vi "convert pixel values to real world.vi"() -> ()   [LabVIEW 2013]
uses:
  <vilib>/vision/Calibration.llb/Calibration Reference Points.ctl
  <vilib>/vision/NI_Vision_Development_Module.lvlib
panel:
  out "manual bottom FangYang vs Ueda":T1[](array[typedef])=[{"X"=365.0, "Y"=447.0}, {"X"=363.0, "Y"=447.0}, {"X"=365.0, "Y"=440.0}, {"X"=360.0, "Y"=440.0}, {"X"=351.0, "Y"=442.0}, {"X"=350.0, "Y"=445.0}, {"X"=347.0, "Y"=443.0}, {"X"=352.0, "Y"=437.0}, {"X"=364.0, "Y"=426.0}, {"X"=392.0, "Y"=419.0}, {"X"=422.0, "Y"=411.0}, {"X"=431.0, "Y"=406.0}, {"X"=441.0, "Y"=402.0}, {"X"=445.0, "Y"=405.0}, {"X"=447.0, "Y"=409.0}, {"X"=452.0, "Y"=407.0}, {"X"=444.0, "Y"=409.0}, {"X"=425.0, "Y"=408.0}, {"X"=410.0, "Y"=416.0}, {"X"=405.0, "Y"=422.0}, {"X"=400.0, "Y"=430.0}, {"X"=400.0, "Y"=423.0}, {"X"=421.0, "Y"=411.0}, {"X"=444.0, "Y"=405.0}, {"X"=451.0, "Y"=407.0}, {"X"=457.0, "Y"=407.0}, {"X"=462.0, "Y"=407.0}, {"X"=463.0, "Y"=406.0}, {"X"=454.0, "Y"=405.0}, {"X"=446.0, "Y"=408.0}, {"X"=435.0, "Y"=414.0}, {"X"=416.0, "Y"=423.0}, {"X"=406.0, "Y"=428.0}, {"X"=399.0, "Y"=438.0}, {"X"=392.0, "Y"=448.0}, {"X"=391.0, "Y"=450.0}, {"X"=387.0, "Y"=448.0}, {"X"=381.0, "Y"=453.0}, {"X"=376.0, "Y"=467.0}, {"X"=370.0, "Y"=469.0}, {"X"=377.0, "Y"=470.0}, {"X"=391.0, "Y"=467.0}, {"X"=412.0, "Y"=468.0}, {"X"=422.0, "Y"=470.0}, {"X"=425.0, "Y"=469.0}, {"X"=426.0, "Y"=466.0}, {"X"=413.0, "Y"=467.0}, {"X"=402.0, "Y"=456.0}, {"X"=384.0, "Y"=452.0}, {"X"=361.0, "Y"=451.0}, {"X"=363.0, "Y"=451.0}, {"X"=353.0, "Y"=456.0}, {"X"=351.0, "Y"=457.0}, {"X"=337.0, "Y"=463.0}, {"X"=324.0, "Y"=475.0}, {"X"=329.0, "Y"=482.0}, {"X"=330.0, "Y"=498.0}, {"X"=333.0, "Y"=505.0}, {"X"=332.0, "Y"=519.0}, {"X"=331.0, "Y"=530.0}, {"X"=328.0, "Y"=526.0}, {"X"=328.0, "Y"=523.0}, {"X"=322.0, "Y"=528.0}, {"X"=316.0, "Y"=530.0}, {"X"=312.0, "Y"=524.0}, {"X"=300.0, "Y"=512.0}, {"X"=296.0, "Y"=507.0}, {"X"=297.0, "Y"=504.0}, {"X"=300.0, "Y"=489.0}, {"X"=300.0, "Y"=484.0}, {"X"=306.0, "Y"=479.0}, {"X"=306.0, "Y"=475.0}, {"X"=306.0, "Y"=466.0}, {"X"=307.0, "Y"=452.0}, {"X"=294.0, "Y"=442.0}, {"X"=266.0, "Y"=436.0}, {"X"=237.0, "Y"=417.0}, {"X"=215.0, "Y"=412.0}, {"X"=208.0, "Y"=420.0}, {"X"=205.0, "Y"=413.0}, {"X"=205.0, "Y"=410.0}, {"X"=206.0, "Y"=413.0}, {"X"=225.0, "Y"=422.0}, {"X"=246.0, "Y"=432.0}, {"X"=249.0, "Y"=435.0}, {"X"=258.0, "Y"=442.0}, {"X"=274.0, "Y"=448.0}, {"X"=285.0, "Y"=455.0}, {"X"=296.0, "Y"=458.0}, {"X"=297.0, "Y"=457.0}, {"X"=283.0, "Y"=455.0}, {"X"=272.0, "Y"=459.0}, {"X"=257.0, "Y"=462.0}, {"X"=250.0, "Y"=470.0}, {"X"=238.0, "Y"=474.0}, {"X"=232.0, "Y"=487.0}, {"X"=223.0, "Y"=494.0}, {"X"=219.0, "Y"=499.0}, {"X"=221.0, "Y"=512.0}, {"X"=214.0, "Y"=514.0}, {"X"=216.0, "Y"=508.0}, {"X"=230.0, "Y"=496.0}, {"X"=245.0, "Y"=485.0}, {"X"=258.0, "Y"=484.0}, {"X"=287.0, "Y"=471.0}, {"X"=310.0, "Y"=461.0}, {"X"=315.0, "Y"=456.0}, {"X"=324.0, "Y"=449.0}, {"X"=330.0, "Y"=437.0}, {"X"=340.0, "Y"=429.0}, {"X"=347.0, "Y"=438.0}, {"X"=354.0, "Y"=446.0}, {"X"=353.0, "Y"=449.0}, {"X"=359.0, "Y"=451.0}, {"X"=368.0, "Y"=445.0}, {"X"=258.0, "Y"=444.0}, {"X"=262.0, "Y"=440.0}, {"X"=272.0, "Y"=434.0}, {"X"=274.0, "Y"=426.0}, {"X"=277.0, "Y"=423.0}, {"X"=276.0, "Y"=426.0}, {"X"=277.0, "Y"=423.0}, {"X"=282.0, "Y"=423.0}, {"X"=285.0, "Y"=426.0}, {"X"=288.0, "Y"=430.0}, {"X"=292.0, "Y"=438.0}, {"X"=293.0, "Y"=446.0}, {"X"=290.0, "Y"=454.0}, {"X"=293.0, "Y"=456.0}, {"X"=299.0, "Y"=464.0}, {"X"=303.0, "Y"=464.0}, {"X"=300.0, "Y"=464.0}, {"X"=294.0, "Y"=464.0}, {"X"=289.0, "Y"=462.0}, {"X"=273.0, "Y"=460.0}, {"X"=245.0, "Y"=457.0}, {"X"=213.0, "Y"=463.0}, {"X"=205.0, "Y"=465.0}, {"X"=205.0, "Y"=463.0}, {"X"=214.0, "Y"=462.0}, {"X"=245.0, "Y"=460.0}, {"X"=287.0, "Y"=466.0}, {"X"=303.0, "Y"=463.0}, {"X"=315.0, "Y"=457.0}, {"X"=335.0, "Y"=469.0}, {"X"=352.0, "Y"=471.0}, {"X"=361.0, "Y"=465.0}, {"X"=366.0, "Y"=466.0}, {"X"=370.0, "Y"=463.0}, {"X"=376.0, "Y"=467.0}, {"X"=373.0, "Y"=466.0}, {"X"=377.0, "Y"=473.0}, {"X"=376.0, "Y"=471.0}, {"X"=358.0, "Y"=474.0}, {"X"=339.0, "Y"=475.0}, {"X"=420.0, "Y"=441.0}, {"X"=420.0, "Y"=443.0}, {"X"=420.0, "Y"=443.0}, {"X"=424.0, "Y"=435.0}, {"X"=431.0, "Y"=430.0}, {"X"=426.0, "Y"=426.0}, {"X"=427.0, "Y"=427.0}, {"X"=425.0, "Y"=425.0}, {"X"=423.0, "Y"=424.0}, {"X"=415.0, "Y"=430.0}, {"X"=417.0, "Y"=432.0}, {"X"=415.0, "Y"=438.0}, {"X"=410.0, "Y"=441.0}, {"X"=399.0, "Y"=450.0}, {"X"=389.0, "Y"=458.0}, {"X"=388.0, "Y"=459.0}, {"X"=400.0, "Y"=461.0}, {"X"=412.0, "Y"=463.0}, {"X"=413.0, "Y"=458.0}, {"X"=413.0, "Y"=458.0}, {"X"=416.0, "Y"=458.0}, {"X"=420.0, "Y"=460.0}, {"X"=419.0, "Y"=459.0}, {"X"=402.0, "Y"=459.0}, {"X"=395.0, "Y"=460.0}, {"X"=394.0, "Y"=459.0}, {"X"=396.0, "Y"=454.0}, {"X"=397.0, "Y"=452.0}, {"X"=396.0, "Y"=451.0}, {"X"=401.0, "Y"=454.0}, {"X"=408.0, "Y"=442.0}, {"X"=410.0, "Y"=428.0}, {"X"=411.0, "Y"=417.0}, {"X"=404.0, "Y"=402.0}, {"X"=405.0, "Y"=403.0}, {"X"=404.0, "Y"=405.0}, {"X"=396.0, "Y"=402.0}, {"X"=387.0, "Y"=406.0}, {"X"=382.0, "Y"=408.0}, {"X"=378.0, "Y"=413.0}, {"X"=361.0, "Y"=417.0}, {"X"=346.0, "Y"=433.0}, {"X"=335.0, "Y"=443.0}, {"X"=329.0, "Y"=445.0}, {"X"=317.0, "Y"=452.0}, {"X"=313.0, "Y"=457.0}, {"X"=312.0, "Y"=465.0}, {"X"=309.0, "Y"=467.0}, {"X"=305.0, "Y"=469.0}, {"X"=298.0, "Y"=463.0}, {"X"=292.0, "Y"=463.0}, {"X"=267.0, "Y"=466.0}, {"X"=267.0, "Y"=464.0}, {"X"=266.0, "Y"=467.0}, {"X"=268.0, "Y"=465.0}, {"X"=284.0, "Y"=467.0}, {"X"=296.0, "Y"=464.0}, {"X"=303.0, "Y"=466.0}, {"X"=310.0, "Y"=466.0}, {"X"=318.0, "Y"=464.0}, {"X"=327.0, "Y"=467.0}, {"X"=322.0, "Y"=466.0}, {"X"=318.0, "Y"=462.0}, {"X"=297.0, "Y"=465.0}, {"X"=263.0, "Y"=468.0}, {"X"=222.0, "Y"=468.0}, {"X"=174.0, "Y"=472.0}, {"X"=142.0, "Y"=470.0}, {"X"=130.0, "Y"=467.0}, {"X"=131.0, "Y"=467.0}, {"X"=157.0, "Y"=461.0}, {"X"=177.0, "Y"=459.0}, {"X"=207.0, "Y"=458.0}, {"X"=248.0, "Y"=459.0}, {"X"=276.0, "Y"=464.0}, {"X"=300.0, "Y"=463.0}, {"X"=318.0, "Y"=457.0}, {"X"=257.0, "Y"=443.0}, {"X"=260.0, "Y"=444.0}, {"X"=260.0, "Y"=439.0}, {"X"=263.0, "Y"=435.0}, {"X"=268.0, "Y"=424.0}, {"X"=275.0, "Y"=426.0}, {"X"=281.0, "Y"=424.0}, {"X"=278.0, "Y"=415.0}, {"X"=286.0, "Y"=421.0}, {"X"=283.0, "Y"=422.0}, {"X"=289.0, "Y"=416.0}, {"X"=289.0, "Y"=417.0}, {"X"=293.0, "Y"=420.0}, {"X"=290.0, "Y"=423.0}, {"X"=295.0, "Y"=423.0}, {"X"=304.0, "Y"=430.0}, {"X"=304.0, "Y"=441.0}, {"X"=318.0, "Y"=454.0}, {"X"=325.0, "Y"=464.0}, {"X"=334.0, "Y"=469.0}, {"X"=360.0, "Y"=488.0}, {"X"=387.0, "Y"=497.0}, {"X"=409.0, "Y"=511.0}, {"X"=428.0, "Y"=520.0}, {"X"=426.0, "Y"=519.0}, {"X"=422.0, "Y"=514.0}, {"X"=406.0, "Y"=509.0}, {"X"=402.0, "Y"=506.0}, {"X"=402.0, "Y"=502.0}, {"X"=402.0, "Y"=491.0}, {"X"=398.0, "Y"=478.0}, {"X"=394.0, "Y"=471.0}, {"X"=375.0, "Y"=463.0}, {"X"=372.0, "Y"=470.0}, {"X"=375.0, "Y"=473.0}, {"X"=374.0, "Y"=475.0}, {"X"=395.0, "Y"=478.0}, {"X"=425.0, "Y"=485.0}, {"X"=458.0, "Y"=501.0}, {"X"=492.0, "Y"=510.0}, {"X"=503.0, "Y"=518.0}, {"X"=492.0, "Y"=514.0}, {"X"=474.0, "Y"=508.0}, {"X"=459.0, "Y"=499.0}, {"X"=449.0, "Y"=502.0}, {"X"=435.0, "Y"=492.0}, {"X"=414.0, "Y"=490.0}, {"X"=385.0, "Y"=473.0}, {"X"=365.0, "Y"=466.0}, {"X"=338.0, "Y"=464.0}, {"X"=329.0, "Y"=464.0}, {"X"=330.0, "Y"=469.0}, {"X"=334.0, "Y"=476.0}, {"X"=348.0, "Y"=483.0}, {"X"=379.0, "Y"=487.0}, {"X"=405.0, "Y"=495.0}, {"X"=442.0, "Y"=501.0}, {"X"=466.0, "Y"=512.0}, {"X"=476.0, "Y"=515.0}, {"X"=474.0, "Y"=515.0}, {"X"=452.0, "Y"=502.0}, {"X"=435.0, "Y"=497.0}, {"X"=437.0, "Y"=499.0}, {"X"=426.0, "Y"=491.0}, {"X"=415.0, "Y"=481.0}, {"X"=407.0, "Y"=469.0}, {"X"=398.0, "Y"=466.0}, {"X"=384.0, "Y"=465.0}, {"X"=377.0, "Y"=466.0}, {"X"=363.0, "Y"=467.0}, {"X"=329.0, "Y"=475.0}, {"X"=305.0, "Y"=482.0}, {"X"=281.0, "Y"=492.0}, {"X"=252.0, "Y"=507.0}, {"X"=231.0, "Y"=504.0}, {"X"=212.0, "Y"=508.0}, {"X"=203.0, "Y"=516.0}, {"X"=189.0, "Y"=515.0}, {"X"=196.0, "Y"=511.0}, {"X"=221.0, "Y"=496.0}, {"X"=229.0, "Y"=491.0}, {"X"=227.0, "Y"=488.0}, {"X"=223.0, "Y"=483.0}, {"X"=224.0, "Y"=473.0}, {"X"=429.0, "Y"=442.0}, {"X"=430.0, "Y"=440.0}, {"X"=428.0, "Y"=432.0}, {"X"=431.0, "Y"=434.0}, {"X"=425.0, "Y"=430.0}, {"X"=419.0, "Y"=430.0}, {"X"=411.0, "Y"=429.0}, {"X"=411.0, "Y"=430.0}, {"X"=394.0, "Y"=435.0}, {"X"=377.0, "Y"=438.0}, {"X"=357.0, "Y"=447.0}, {"X"=346.0, "Y"=450.0}, {"X"=329.0, "Y"=448.0}, {"X"=319.0, "Y"=458.0}, {"X"=303.0, "Y"=460.0}, {"X"=306.0, "Y"=458.0}, {"X"=285.0, "Y"=459.0}, {"X"=262.0, "Y"=460.0}, {"X"=243.0, "Y"=471.0}, {"X"=222.0, "Y"=481.0}, {"X"=201.0, "Y"=484.0}, {"X"=184.0, "Y"=493.0}, {"X"=170.0, "Y"=504.0}, {"X"=160.0, "Y"=512.0}, {"X"=147.0, "Y"=519.0}, {"X"=155.0, "Y"=519.0}, {"X"=180.0, "Y"=512.0}, {"X"=206.0, "Y"=505.0}, {"X"=213.0, "Y"=501.0}, {"X"=226.0, "Y"=489.0}, {"X"=243.0, "Y"=482.0}, {"X"=255.0, "Y"=475.0}, {"X"=260.0, "Y"=469.0}, {"X"=274.0, "Y"=464.0}, {"X"=285.0, "Y"=466.0}, {"X"=280.0, "Y"=463.0}, {"X"=271.0, "Y"=464.0}, {"X"=247.0, "Y"=464.0}, {"X"=225.0, "Y"=473.0}, {"X"=218.0, "Y"=485.0}, {"X"=197.0, "Y"=496.0}, {"X"=191.0, "Y"=485.0}, {"X"=183.0, "Y"=496.0}, {"X"=188.0, "Y"=500.0}, {"X"=166.0, "Y"=520.0}, {"X"=170.0, "Y"=514.0}, {"X"=172.0, "Y"=512.0}, {"X"=184.0, "Y"=508.0}, {"X"=200.0, "Y"=501.0}, {"X"=241.0, "Y"=486.0}, {"X"=271.0, "Y"=473.0}, {"X"=326.0, "Y"=446.0}, {"X"=335.0, "Y"=448.0}, {"X"=334.0, "Y"=446.0}, {"X"=360.0, "Y"=444.0}, {"X"=375.0, "Y"=447.0}, {"X"=380.0, "Y"=443.0}, {"X"=386.0, "Y"=430.0}, {"X"=386.0, "Y"=424.0}, {"X"=389.0, "Y"=407.0}, {"X"=385.0, "Y"=400.0}, {"X"=387.0, "Y"=396.0}, {"X"=381.0, "Y"=400.0}, {"X"=380.0, "Y"=404.0}, {"X"=379.0, "Y"=407.0}, {"X"=355.0, "Y"=423.0}, {"X"=340.0, "Y"=430.0}, {"X"=331.0, "Y"=437.0}, {"X"=317.0, "Y"=439.0}, {"X"=308.0, "Y"=447.0}, {"X"=284.0, "Y"=454.0}, {"X"=279.0, "Y"=456.0}, {"X"=266.0, "Y"=458.0}, {"X"=262.0, "Y"=459.0}, {"X"=258.0, "Y"=459.0}, {"X"=237.0, "Y"=452.0}, {"X"=231.0, "Y"=449.0}, {"X"=239.0, "Y"=448.0}, {"X"=250.0, "Y"=451.0}, {"X"=264.0, "Y"=450.0}, {"X"=290.0, "Y"=450.0}, {"X"=315.0, "Y"=449.0}, {"X"=329.0, "Y"=453.0}, {"X"=340.0, "Y"=452.0}, {"X"=363.0, "Y"=447.0}, {"X"=382.0, "Y"=432.0}, {"X"=396.0, "Y"=421.0}, {"X"=404.0, "Y"=408.0}, {"X"=408.0, "Y"=407.0}, {"X"=420.0, "Y"=401.0}, {"X"=416.0, "Y"=395.0}, {"X"=418.0, "Y"=400.0}, {"X"=413.0, "Y"=403.0}, {"X"=397.0, "Y"=416.0}, {"X"=393.0, "Y"=418.0}, {"X"=384.0, "Y"=427.0}, {"X"=382.0, "Y"=431.0}, {"X"=380.0, "Y"=435.0}, {"X"=381.0, "Y"=445.0}, {"X"=388.0, "Y"=450.0}, {"X"=382.0, "Y"=460.0}, {"X"=400.0, "Y"=455.0}, {"X"=436.0, "Y"=457.0}, {"X"=456.0, "Y"=449.0}, {"X"=468.0, "Y"=450.0}, {"X"=477.0, "Y"=450.0}, {"X"=474.0, "Y"=448.0}, {"X"=461.0, "Y"=450.0}, {"X"=457.0, "Y"=451.0}, {"X"=451.0, "Y"=445.0}, {"X"=436.0, "Y"=444.0}, {"X"=414.0, "Y"=446.0}, {"X"=391.0, "Y"=445.0}, {"X"=372.0, "Y"=453.0}, {"X"=364.0, "Y"=447.0}, {"X"=363.0, "Y"=454.0}, {"X"=358.0, "Y"=464.0}, {"X"=358.0, "Y"=472.0}, {"X"=373.0, "Y"=484.0}, {"X"=396.0, "Y"=493.0}, {"X"=415.0, "Y"=477.0}, {"X"=439.0, "Y"=502.0}, {"X"=472.0, "Y"=519.0}, {"X"=508.0, "Y"=541.0}, {"X"=497.0, "Y"=529.0}, {"X"=486.0, "Y"=519.0}, {"X"=471.0, "Y"=511.0}, {"X"=452.0, "Y"=501.0}, {"X"=440.0, "Y"=488.0}, {"X"=428.0, "Y"=475.0}, {"X"=404.0, "Y"=462.0}, {"X"=393.0, "Y"=441.0}, {"X"=379.0, "Y"=433.0}, {"X"=381.0, "Y"=437.0}, {"X"=383.0, "Y"=432.0}, {"X"=376.0, "Y"=428.0}, {"X"=370.0, "Y"=429.0}, {"X"=364.0, "Y"=431.0}, {"X"=369.0, "Y"=438.0}, {"X"=364.0, "Y"=442.0}, {"X"=363.0, "Y"=447.0}, {"X"=360.0, "Y"=450.0}, {"X"=360.0, "Y"=457.0}, {"X"=370.0, "Y"=461.0}, {"X"=374.0, "Y"=466.0}, {"X"=371.0, "Y"=466.0}, {"X"=360.0, "Y"=461.0}, {"X"=332.0, "Y"=465.0}, {"X"=299.0, "Y"=453.0}, {"X"=266.0, "Y"=435.0}, {"X"=250.0, "Y"=439.0}, {"X"=236.0, "Y"=435.0}, {"X"=229.0, "Y"=424.0}, {"X"=228.0, "Y"=431.0}, {"X"=232.0, "Y"=440.0}, {"X"=235.0, "Y"=447.0}, {"X"=252.0, "Y"=452.0}, {"X"=265.0, "Y"=462.0}, {"X"=275.0, "Y"=463.0}, {"X"=266.0, "Y"=465.0}, {"X"=269.0, "Y"=466.0}, {"X"=270.0, "Y"=465.0}, {"X"=263.0, "Y"=463.0}, {"X"=266.0, "Y"=467.0}, {"X"=268.0, "Y"=464.0}, {"X"=287.0, "Y"=461.0}, {"X"=312.0, "Y"=460.0}, {"X"=334.0, "Y"=466.0}, {"X"=339.0, "Y"=462.0}, {"X"=342.0, "Y"=463.0}, {"X"=329.0, "Y"=469.0}, {"X"=304.0, "Y"=477.0}, {"X"=290.0, "Y"=489.0}, {"X"=266.0, "Y"=493.0}, {"X"=235.0, "Y"=493.0}, {"X"=215.0, "Y"=498.0}, {"X"=200.0, "Y"=509.0}, {"X"=170.0, "Y"=522.0}, {"X"=166.0, "Y"=526.0}, {"X"=175.0, "Y"=521.0}, {"X"=203.0, "Y"=501.0}, {"X"=232.0, "Y"=491.0}, {"X"=256.0, "Y"=495.0}, {"X"=259.0, "Y"=481.0}, {"X"=254.0, "Y"=469.0}, {"X"=251.0, "Y"=449.0}, {"X"=240.0, "Y"=443.0}, {"X"=228.0, "Y"=434.0}, {"X"=224.0, "Y"=422.0}, {"X"=219.0, "Y"=413.0}, {"X"=207.0, "Y"=413.0}, {"X"=419.0, "Y"=440.0}, {"X"=422.0, "Y"=437.0}, {"X"=416.0, "Y"=436.0}, {"X"=429.0, "Y"=444.0}, {"X"=436.0, "Y"=452.0}, {"X"=437.0, "Y"=457.0}, {"X"=449.0, "Y"=468.0}, {"X"=460.0, "Y"=483.0}, {"X"=468.0, "Y"=496.0}, {"X"=478.0, "Y"=508.0}, {"X"=467.0, "Y"=503.0}, {"X"=438.0, "Y"=493.0}, {"X"=434.0, "Y"=496.0}, {"X"=427.0, "Y"=491.0}, {"X"=416.0, "Y"=481.0}, {"X"=402.0, "Y"=473.0}, {"X"=399.0, "Y"=469.0}, {"X"=405.0, "Y"=458.0}, {"X"=394.0, "Y"=446.0}, {"X"=374.0, "Y"=435.0}, {"X"=359.0, "Y"=429.0}, {"X"=350.0, "Y"=422.0}, {"X"=347.0, "Y"=421.0}, {"X"=338.0, "Y"=426.0}, {"X"=329.0, "Y"=426.0}, {"X"=327.0, "Y"=427.0}, {"X"=326.0, "Y"=426.0}, {"X"=340.0, "Y"=433.0}, {"X"=345.0, "Y"=432.0}, {"X"=379.0, "Y"=421.0}, {"X"=403.0, "Y"=415.0}, {"X"=403.0, "Y"=419.0}, {"X"=411.0, "Y"=413.0}, {"X"=409.0, "Y"=404.0}, {"X"=413.0, "Y"=391.0}, {"X"=403.0, "Y"=377.0}, {"X"=405.0, "Y"=377.0}, {"X"=409.0, "Y"=370.0}, {"X"=412.0, "Y"=366.0}, {"X"=397.0, "Y"=370.0}, {"X"=376.0, "Y"=376.0}, {"X"=366.0, "Y"=377.0}, {"X"=348.0, "Y"=376.0}, {"X"=0.0, "Y"=0.0}] {"Y" format="%.2f"; "X" format="%.2f"}
  in  "auto top FangYang vs Ueda":cluster{"Numeric":dbl, "Numeric":dbl}[](array[cluster])=[{"Numeric"=0.0, "Numeric"=0.0}, {"Numeric"=288.0, "Numeric"=288.0}, {"Numeric"=285.0, "Numeric"=292.0}, {"Numeric"=286.0, "Numeric"=308.0}, {"Numeric"=292.0, "Numeric"=309.0}, {"Numeric"=307.0, "Numeric"=306.0}, {"Numeric"=311.0, "Numeric"=298.0}, {"Numeric"=316.0, "Numeric"=299.0}, {"Numeric"=324.0, "Numeric"=289.0}, {"Numeric"=332.0, "Numeric"=288.0}, {"Numeric"=336.0, "Numeric"=294.0}, {"Numeric"=355.0, "Numeric"=288.0}, {"Numeric"=374.0, "Numeric"=286.0}, {"Numeric"=381.0, "Numeric"=288.0}, {"Numeric"=381.0, "Numeric"=288.0}, {"Numeric"=420.0, "Numeric"=295.0}, {"Numeric"=426.0, "Numeric"=296.0}, {"Numeric"=442.0, "Numeric"=308.0}, {"Numeric"=456.0, "Numeric"=318.0}, {"Numeric"=465.0, "Numeric"=330.0}, {"Numeric"=470.0, "Numeric"=321.0}, {"Numeric"=457.0, "Numeric"=312.0}, {"Numeric"=457.0, "Numeric"=312.0}, {"Numeric"=448.0, "Numeric"=310.0}, {"Numeric"=443.0, "Numeric"=295.0}, {"Numeric"=437.0, "Numeric"=291.0}, {"Numeric"=421.0, "Numeric"=295.0}, {"Numeric"=408.0, "Numeric"=298.0}, {"Numeric"=402.0, "Numeric"=298.0}, {"Numeric"=380.0, "Numeric"=298.0}, {"Numeric"=380.0, "Numeric"=277.0}, {"Numeric"=407.0, "Numeric"=299.0}, {"Numeric"=410.0, "Numeric"=299.0}, {"Numeric"=418.0, "Numeric"=257.0}, {"Numeric"=430.0, "Numeric"=252.0}, {"Numeric"=436.0, "Numeric"=252.0}, {"Numeric"=446.0, "Numeric"=242.0}, {"Numeric"=444.0, "Numeric"=236.0}, {"Numeric"=448.0, "Numeric"=230.0}, {"Numeric"=448.0, "Numeric"=234.0}, {"Numeric"=451.0, "Numeric"=236.0}, {"Numeric"=452.0, "Numeric"=243.0}, {"Numeric"=450.0, "Numeric"=254.0}, {"Numeric"=446.0, "Numeric"=263.0}, {"Numeric"=440.0, "Numeric"=272.0}, {"Numeric"=435.0, "Numeric"=273.0}, {"Numeric"=426.0, "Numeric"=281.0}, {"Numeric"=426.0, "Numeric"=290.0}, {"Numeric"=418.0, "Numeric"=292.0}, {"Numeric"=410.0, "Numeric"=318.0}, {"Numeric"=400.0, "Numeric"=331.0}, {"Numeric"=392.0, "Numeric"=336.0}, {"Numeric"=373.0, "Numeric"=309.0}, {"Numeric"=370.0, "Numeric"=312.0}, {"Numeric"=371.0, "Numeric"=313.0}, {"Numeric"=371.0, "Numeric"=299.0}, {"Numeric"=368.0, "Numeric"=298.0}, {"Numeric"=369.0, "Numeric"=297.0}, {"Numeric"=364.0, "Numeric"=292.0}, {"Numeric"=358.0, "Numeric"=283.0}, {"Numeric"=352.0, "Numeric"=278.0}, {"Numeric"=350.0, "Numeric"=278.0}, {"Numeric"=349.0, "Numeric"=276.0}, {"Numeric"=342.0, "Numeric"=273.0}, {"Numeric"=329.0, "Numeric"=270.0}, {"Numeric"=328.0, "Numeric"=270.0}, {"Numeric"=330.0, "Numeric"=269.0}, {"Numeric"=316.0, "Numeric"=271.0}, {"Numeric"=289.0, "Numeric"=268.0}, {"Numeric"=270.0, "Numeric"=282.0}, {"Numeric"=265.0, "Numeric"=286.0}, {"Numeric"=262.0, "Numeric"=263.0}, {"Numeric"=256.0, "Numeric"=281.0}, {"Numeric"=258.0, "Numeric"=282.0}, {"Numeric"=262.0, "Numeric"=278.0}, {"Numeric"=269.0, "Numeric"=289.0}, {"Numeric"=277.0, "Numeric"=289.0}, {"Numeric"=271.0, "Numeric"=288.0}, {"Numeric"=278.0, "Numeric"=287.0}, {"Numeric"=286.0, "Numeric"=284.0}, {"Numeric"=290.0, "Numeric"=284.0}, {"Numeric"=277.0, "Numeric"=283.0}, {"Numeric"=277.0, "Numeric"=272.0}, {"Numeric"=282.0, "Numeric"=268.0}, {"Numeric"=274.0, "Numeric"=265.0}, {"Numeric"=265.0, "Numeric"=255.0}, {"Numeric"=269.0, "Numeric"=253.0}, {"Numeric"=253.0, "Numeric"=235.0}, {"Numeric"=248.0, "Numeric"=231.0}, {"Numeric"=249.0, "Numeric"=235.0}, {"Numeric"=257.0, "Numeric"=238.0}, {"Numeric"=260.0, "Numeric"=240.0}, {"Numeric"=268.0, "Numeric"=249.0}, {"Numeric"=275.0, "Numeric"=253.0}, {"Numeric"=283.0, "Numeric"=257.0}, {"Numeric"=287.0, "Numeric"=263.0}, {"Numeric"=293.0, "Numeric"=263.0}, {"Numeric"=302.0, "Numeric"=266.0}, {"Numeric"=303.0, "Numeric"=271.0}, {"Numeric"=301.0, "Numeric"=271.0}, {"Numeric"=290.0, "Numeric"=272.0}, {"Numeric"=296.0, "Numeric"=249.0}, {"Numeric"=299.0, "Numeric"=269.0}, {"Numeric"=304.0, "Numeric"=267.0}, {"Numeric"=312.0, "Numeric"=271.0}, {"Numeric"=316.0, "Numeric"=271.0}, {"Numeric"=319.0, "Numeric"=271.0}, {"Numeric"=322.0, "Numeric"=271.0}, {"Numeric"=312.0, "Numeric"=270.0}, {"Numeric"=337.0, "Numeric"=269.0}, {"Numeric"=335.0, "Numeric"=275.0}, {"Numeric"=367.0, "Numeric"=270.0}, {"Numeric"=328.0, "Numeric"=273.0}, {"Numeric"=380.0, "Numeric"=274.0}, {"Numeric"=374.0, "Numeric"=274.0}, {"Numeric"=374.0, "Numeric"=274.0}, {"Numeric"=340.0, "Numeric"=286.0}, {"Numeric"=336.0, "Numeric"=287.0}, {"Numeric"=336.0, "Numeric"=281.0}, {"Numeric"=336.0, "Numeric"=285.0}, {"Numeric"=333.0, "Numeric"=285.0}, {"Numeric"=335.0, "Numeric"=284.0}, {"Numeric"=334.0, "Numeric"=285.0}, {"Numeric"=328.0, "Numeric"=295.0}, {"Numeric"=307.0, "Numeric"=284.0}, {"Numeric"=280.0, "Numeric"=283.0}, {"Numeric"=276.0, "Numeric"=283.0}, {"Numeric"=274.0, "Numeric"=267.0}, {"Numeric"=264.0, "Numeric"=250.0}, {"Numeric"=259.0, "Numeric"=249.0}, {"Numeric"=244.0, "Numeric"=243.0}, {"Numeric"=234.0, "Numeric"=232.0}, {"Numeric"=247.0, "Numeric"=241.0}, {"Numeric"=251.0, "Numeric"=241.0}, {"Numeric"=267.0, "Numeric"=251.0}, {"Numeric"=280.0, "Numeric"=262.0}, {"Numeric"=289.0, "Numeric"=272.0}, {"Numeric"=307.0, "Numeric"=258.0}, {"Numeric"=319.0, "Numeric"=283.0}, {"Numeric"=340.0, "Numeric"=283.0}, {"Numeric"=374.0, "Numeric"=299.0}, {"Numeric"=387.0, "Numeric"=307.0}, {"Numeric"=375.0, "Numeric"=301.0}, {"Numeric"=403.0, "Numeric"=313.0}, {"Numeric"=415.0, "Numeric"=312.0}, {"Numeric"=409.0, "Numeric"=307.0}, {"Numeric"=361.0, "Numeric"=311.0}, {"Numeric"=411.0, "Numeric"=313.0}, {"Numeric"=419.0, "Numeric"=312.0}, {"Numeric"=444.0, "Numeric"=310.0}, {"Numeric"=436.0, "Numeric"=325.0}, {"Numeric"=442.0, "Numeric"=328.0}, {"Numeric"=446.0, "Numeric"=325.0}, {"Numeric"=447.0, "Numeric"=332.0}, {"Numeric"=449.0, "Numeric"=340.0}, {"Numeric"=449.0, "Numeric"=340.0}, {"Numeric"=333.0, "Numeric"=275.0}, {"Numeric"=335.0, "Numeric"=281.0}, {"Numeric"=336.0, "Numeric"=276.0}, {"Numeric"=334.0, "Numeric"=277.0}, {"Numeric"=341.0, "Numeric"=283.0}, {"Numeric"=352.0, "Numeric"=288.0}, {"Numeric"=360.0, "Numeric"=285.0}, {"Numeric"=367.0, "Numeric"=282.0}, {"Numeric"=378.0, "Numeric"=288.0}, {"Numeric"=386.0, "Numeric"=270.0}, {"Numeric"=388.0, "Numeric"=266.0}, {"Numeric"=403.0, "Numeric"=261.0}, {"Numeric"=407.0, "Numeric"=257.0}, {"Numeric"=419.0, "Numeric"=255.0}, {"Numeric"=429.0, "Numeric"=253.0}, {"Numeric"=436.0, "Numeric"=258.0}, {"Numeric"=409.0, "Numeric"=261.0}, {"Numeric"=401.0, "Numeric"=258.0}, {"Numeric"=392.0, "Numeric"=263.0}, {"Numeric"=381.0, "Numeric"=273.0}, {"Numeric"=377.0, "Numeric"=277.0}, {"Numeric"=371.0, "Numeric"=276.0}, {"Numeric"=377.0, "Numeric"=281.0}, {"Numeric"=388.0, "Numeric"=281.0}, {"Numeric"=413.0, "Numeric"=288.0}, {"Numeric"=432.0, "Numeric"=288.0}, {"Numeric"=435.0, "Numeric"=296.0}, {"Numeric"=456.0, "Numeric"=310.0}, {"Numeric"=453.0, "Numeric"=320.0}, {"Numeric"=450.0, "Numeric"=316.0}, {"Numeric"=450.0, "Numeric"=316.0}, {"Numeric"=433.0, "Numeric"=320.0}, {"Numeric"=426.0, "Numeric"=314.0}, {"Numeric"=405.0, "Numeric"=312.0}, {"Numeric"=406.0, "Numeric"=312.0}, {"Numeric"=392.0, "Numeric"=314.0}, {"Numeric"=379.0, "Numeric"=311.0}, {"Numeric"=359.0, "Numeric"=310.0}, {"Numeric"=342.0, "Numeric"=310.0}, {"Numeric"=334.0, "Numeric"=309.0}, {"Numeric"=309.0, "Numeric"=251.0}, {"Numeric"=333.0, "Numeric"=258.0}, {"Numeric"=313.0, "Numeric"=248.0}, {"Numeric"=291.0, "Numeric"=246.0}, {"Numeric"=277.0, "Numeric"=244.0}, {"Numeric"=265.0, "Numeric"=238.0}, {"Numeric"=267.0, "Numeric"=241.0}, {"Numeric"=270.0, "Numeric"=240.0}, {"Numeric"=277.0, "Numeric"=251.0}, {"Numeric"=291.0, "Numeric"=262.0}, {"Numeric"=293.0, "Numeric"=267.0}, {"Numeric"=294.0, "Numeric"=270.0}, {"Numeric"=288.0, "Numeric"=270.0}, {"Numeric"=275.0, "Numeric"=266.0}, {"Numeric"=272.0, "Numeric"=260.0}, {"Numeric"=271.0, "Numeric"=262.0}, {"Numeric"=274.0, "Numeric"=253.0}, {"Numeric"=266.0, "Numeric"=246.0}, {"Numeric"=265.0, "Numeric"=242.0}, {"Numeric"=260.0, "Numeric"=238.0}, {"Numeric"=260.0, "Numeric"=235.0}, {"Numeric"=261.0, "Numeric"=235.0}, {"Numeric"=260.0, "Numeric"=237.0}, {"Numeric"=258.0, "Numeric"=246.0}, {"Numeric"=264.0, "Numeric"=252.0}, {"Numeric"=263.0, "Numeric"=260.0}, {"Numeric"=259.0, "Numeric"=259.0}, {"Numeric"=252.0, "Numeric"=279.0}, {"Numeric"=247.0, "Numeric"=295.0}, {"Numeric"=238.0, "Numeric"=298.0}, {"Numeric"=233.0, "Numeric"=310.0}, {"Numeric"=225.0, "Numeric"=313.0}, {"Numeric"=228.0, "Numeric"=314.0}, {"Numeric"=196.0, "Numeric"=327.0}, {"Numeric"=192.0, "Numeric"=334.0}, {"Numeric"=184.0, "Numeric"=342.0}, {"Numeric"=182.0, "Numeric"=341.0}, {"Numeric"=339.0, "Numeric"=272.0}, {"Numeric"=340.0, "Numeric"=288.0}, {"Numeric"=346.0, "Numeric"=288.0}, {"Numeric"=344.0, "Numeric"=288.0}, {"Numeric"=335.0, "Numeric"=287.0}, {"Numeric"=335.0, "Numeric"=287.0}, {"Numeric"=330.0, "Numeric"=287.0}, {"Numeric"=305.0, "Numeric"=295.0}, {"Numeric"=289.0, "Numeric"=292.0}, {"Numeric"=292.0, "Numeric"=296.0}, {"Numeric"=278.0, "Numeric"=301.0}, {"Numeric"=257.0, "Numeric"=315.0}, {"Numeric"=328.0, "Numeric"=282.0}, {"Numeric"=255.0, "Numeric"=329.0}, {"Numeric"=273.0, "Numeric"=314.0}, {"Numeric"=282.0, "Numeric"=300.0}, {"Numeric"=295.0, "Numeric"=289.0}, {"Numeric"=306.0, "Numeric"=286.0}, {"Numeric"=308.0, "Numeric"=286.0}, {"Numeric"=325.0, "Numeric"=296.0}, {"Numeric"=331.0, "Numeric"=292.0}, {"Numeric"=342.0, "Numeric"=289.0}, {"Numeric"=357.0, "Numeric"=283.0}, {"Numeric"=367.0, "Numeric"=281.0}, {"Numeric"=367.0, "Numeric"=276.0}, {"Numeric"=385.0, "Numeric"=268.0}, {"Numeric"=392.0, "Numeric"=279.0}, {"Numeric"=410.0, "Numeric"=287.0}, {"Numeric"=418.0, "Numeric"=294.0}, {"Numeric"=425.0, "Numeric"=299.0}, {"Numeric"=427.0, "Numeric"=266.0}, {"Numeric"=425.0, "Numeric"=266.0}, {"Numeric"=420.0, "Numeric"=294.0}, {"Numeric"=415.0, "Numeric"=293.0}, {"Numeric"=408.0, "Numeric"=290.0}, {"Numeric"=403.0, "Numeric"=288.0}, {"Numeric"=397.0, "Numeric"=286.0}, {"Numeric"=389.0, "Numeric"=275.0}, {"Numeric"=388.0, "Numeric"=275.0}, {"Numeric"=382.0, "Numeric"=272.0}, {"Numeric"=381.0, "Numeric"=271.0}, {"Numeric"=365.0, "Numeric"=267.0}, {"Numeric"=353.0, "Numeric"=269.0}, {"Numeric"=333.0, "Numeric"=281.0}, {"Numeric"=313.0, "Numeric"=277.0}, {"Numeric"=304.0, "Numeric"=286.0}, {"Numeric"=279.0, "Numeric"=296.0}, {"Numeric"=274.0, "Numeric"=289.0}, {"Numeric"=274.0, "Numeric"=283.0}, {"Numeric"=270.0, "Numeric"=292.0}, {"Numeric"=276.0, "Numeric"=290.0}, {"Numeric"=285.0, "Numeric"=289.0}, {"Numeric"=301.0, "Numeric"=286.0}, {"Numeric"=319.0, "Numeric"=279.0}, {"Numeric"=329.0, "Numeric"=278.0}, {"Numeric"=336.0, "Numeric"=275.0}, {"Numeric"=337.0, "Numeric"=274.0}, {"Numeric"=362.0, "Numeric"=271.0}, {"Numeric"=367.0, "Numeric"=269.0}, {"Numeric"=374.0, "Numeric"=265.0}, {"Numeric"=377.0, "Numeric"=273.0}, {"Numeric"=383.0, "Numeric"=268.0}, {"Numeric"=397.0, "Numeric"=284.0}, {"Numeric"=421.0, "Numeric"=285.0}, {"Numeric"=418.0, "Numeric"=285.0}, {"Numeric"=428.0, "Numeric"=276.0}, {"Numeric"=415.0, "Numeric"=285.0}, {"Numeric"=404.0, "Numeric"=289.0}, {"Numeric"=398.0, "Numeric"=288.0}, {"Numeric"=390.0, "Numeric"=284.0}, {"Numeric"=377.0, "Numeric"=283.0}, {"Numeric"=362.0, "Numeric"=280.0}, {"Numeric"=350.0, "Numeric"=276.0}, {"Numeric"=340.0, "Numeric"=274.0}, {"Numeric"=333.0, "Numeric"=275.0}, {"Numeric"=323.0, "Numeric"=270.0}, {"Numeric"=323.0, "Numeric"=269.0}, {"Numeric"=306.0, "Numeric"=269.0}, {"Numeric"=297.0, "Numeric"=265.0}, {"Numeric"=284.0, "Numeric"=267.0}, {"Numeric"=272.0, "Numeric"=271.0}, {"Numeric"=241.0, "Numeric"=271.0}, {"Numeric"=236.0, "Numeric"=270.0}, {"Numeric"=230.0, "Numeric"=271.0}, {"Numeric"=336.0, "Numeric"=273.0}, {"Numeric"=335.0, "Numeric"=276.0}, {"Numeric"=342.0, "Numeric"=272.0}, {"Numeric"=348.0, "Numeric"=288.0}, {"Numeric"=361.0, "Numeric"=289.0}, {"Numeric"=377.0, "Numeric"=291.0}, {"Numeric"=371.0, "Numeric"=295.0}, {"Numeric"=353.0, "Numeric"=289.0}, {"Numeric"=328.0, "Numeric"=288.0}, {"Numeric"=335.0, "Numeric"=268.0}, {"Numeric"=311.0, "Numeric"=260.0}, {"Numeric"=301.0, "Numeric"=251.0}, {"Numeric"=280.0, "Numeric"=247.0}, {"Numeric"=265.0, "Numeric"=238.0}, {"Numeric"=261.0, "Numeric"=237.0}, {"Numeric"=271.0, "Numeric"=248.0}, {"Numeric"=264.0, "Numeric"=246.0}, {"Numeric"=272.0, "Numeric"=253.0}, {"Numeric"=276.0, "Numeric"=252.0}, {"Numeric"=277.0, "Numeric"=255.0}, {"Numeric"=285.0, "Numeric"=262.0}, {"Numeric"=289.0, "Numeric"=268.0}, {"Numeric"=294.0, "Numeric"=279.0}, {"Numeric"=291.0, "Numeric"=279.0}, {"Numeric"=288.0, "Numeric"=276.0}, {"Numeric"=288.0, "Numeric"=273.0}, {"Numeric"=284.0, "Numeric"=276.0}, {"Numeric"=260.0, "Numeric"=273.0}, {"Numeric"=242.0, "Numeric"=260.0}, {"Numeric"=250.0, "Numeric"=268.0}, {"Numeric"=245.0, "Numeric"=255.0}, {"Numeric"=246.0, "Numeric"=248.0}, {"Numeric"=244.0, "Numeric"=244.0}, {"Numeric"=236.0, "Numeric"=232.0}, {"Numeric"=233.0, "Numeric"=228.0}, {"Numeric"=239.0, "Numeric"=235.0}, {"Numeric"=245.0, "Numeric"=238.0}, {"Numeric"=256.0, "Numeric"=247.0}, {"Numeric"=266.0, "Numeric"=251.0}, {"Numeric"=273.0, "Numeric"=252.0}, {"Numeric"=280.0, "Numeric"=258.0}, {"Numeric"=288.0, "Numeric"=263.0}, {"Numeric"=299.0, "Numeric"=265.0}, {"Numeric"=304.0, "Numeric"=271.0}, {"Numeric"=303.0, "Numeric"=268.0}, {"Numeric"=310.0, "Numeric"=266.0}, {"Numeric"=320.0, "Numeric"=266.0}, {"Numeric"=329.0, "Numeric"=267.0}, {"Numeric"=336.0, "Numeric"=264.0}, {"Numeric"=340.0, "Numeric"=270.0}, {"Numeric"=387.0, "Numeric"=285.0}, {"Numeric"=416.0, "Numeric"=288.0}, {"Numeric"=414.0, "Numeric"=309.0}, {"Numeric"=418.0, "Numeric"=319.0}, {"Numeric"=419.0, "Numeric"=313.0}, {"Numeric"=418.0, "Numeric"=320.0}, {"Numeric"=418.0, "Numeric"=326.0}, {"Numeric"=417.0, "Numeric"=326.0}, {"Numeric"=412.0, "Numeric"=325.0}, {"Numeric"=412.0, "Numeric"=324.0}, {"Numeric"=410.0, "Numeric"=326.0}, {"Numeric"=399.0, "Numeric"=331.0}, {"Numeric"=372.0, "Numeric"=325.0}, {"Numeric"=352.0, "Numeric"=317.0}, {"Numeric"=329.0, "Numeric"=316.0}, {"Numeric"=307.0, "Numeric"=315.0}, {"Numeric"=295.0, "Numeric"=315.0}, {"Numeric"=292.0, "Numeric"=258.0}, {"Numeric"=208.0, "Numeric"=198.0}, {"Numeric"=251.0, "Numeric"=248.0}, {"Numeric"=241.0, "Numeric"=244.0}, {"Numeric"=260.0, "Numeric"=252.0}, {"Numeric"=252.0, "Numeric"=251.0}, {"Numeric"=259.0, "Numeric"=258.0}, {"Numeric"=264.0, "Numeric"=262.0}, {"Numeric"=271.0, "Numeric"=262.0}, {"Numeric"=296.0, "Numeric"=269.0}, {"Numeric"=311.0, "Numeric"=288.0}, {"Numeric"=323.0, "Numeric"=293.0}, {"Numeric"=326.0, "Numeric"=307.0}, {"Numeric"=322.0, "Numeric"=300.0}, {"Numeric"=334.0, "Numeric"=325.0}, {"Numeric"=336.0, "Numeric"=311.0}, {"Numeric"=337.0, "Numeric"=305.0}, {"Numeric"=346.0, "Numeric"=307.0}, {"Numeric"=350.0, "Numeric"=300.0}, {"Numeric"=334.0, "Numeric"=308.0}, {"Numeric"=339.0, "Numeric"=303.0}, {"Numeric"=341.0, "Numeric"=299.0}, {"Numeric"=349.0, "Numeric"=296.0}, {"Numeric"=357.0, "Numeric"=286.0}, {"Numeric"=357.0, "Numeric"=301.0}, {"Numeric"=370.0, "Numeric"=302.0}, {"Numeric"=363.0, "Numeric"=269.0}, {"Numeric"=367.0, "Numeric"=258.0}, {"Numeric"=380.0, "Numeric"=252.0}, {"Numeric"=398.0, "Numeric"=248.0}, {"Numeric"=403.0, "Numeric"=249.0}, {"Numeric"=425.0, "Numeric"=242.0}, {"Numeric"=429.0, "Numeric"=241.0}, {"Numeric"=418.0, "Numeric"=242.0}, {"Numeric"=403.0, "Numeric"=249.0}, {"Numeric"=391.0, "Numeric"=251.0}, {"Numeric"=385.0, "Numeric"=253.0}, {"Numeric"=379.0, "Numeric"=260.0}, {"Numeric"=373.0, "Numeric"=265.0}, {"Numeric"=374.0, "Numeric"=267.0}, {"Numeric"=378.0, "Numeric"=270.0}, {"Numeric"=389.0, "Numeric"=275.0}, {"Numeric"=409.0, "Numeric"=275.0}, {"Numeric"=410.0, "Numeric"=275.0}, {"Numeric"=416.0, "Numeric"=277.0}, {"Numeric"=421.0, "Numeric"=289.0}, {"Numeric"=412.0, "Numeric"=290.0}, {"Numeric"=408.0, "Numeric"=304.0}, {"Numeric"=403.0, "Numeric"=301.0}, {"Numeric"=400.0, "Numeric"=294.0}, {"Numeric"=395.0, "Numeric"=290.0}, {"Numeric"=384.0, "Numeric"=282.0}, {"Numeric"=378.0, "Numeric"=280.0}, {"Numeric"=376.0, "Numeric"=277.0}, {"Numeric"=368.0, "Numeric"=272.0}, {"Numeric"=365.0, "Numeric"=268.0}, {"Numeric"=376.0, "Numeric"=266.0}, {"Numeric"=388.0, "Numeric"=264.0}, {"Numeric"=386.0, "Numeric"=266.0}, {"Numeric"=372.0, "Numeric"=244.0}, {"Numeric"=378.0, "Numeric"=268.0}, {"Numeric"=377.0, "Numeric"=270.0}, {"Numeric"=372.0, "Numeric"=270.0}, {"Numeric"=364.0, "Numeric"=286.0}, {"Numeric"=357.0, "Numeric"=288.0}, {"Numeric"=356.0, "Numeric"=274.0}, {"Numeric"=349.0, "Numeric"=276.0}, {"Numeric"=350.0, "Numeric"=274.0}, {"Numeric"=354.0, "Numeric"=280.0}, {"Numeric"=349.0, "Numeric"=280.0}, {"Numeric"=357.0, "Numeric"=280.0}, {"Numeric"=384.0, "Numeric"=263.0}, {"Numeric"=394.0, "Numeric"=259.0}, {"Numeric"=412.0, "Numeric"=255.0}, {"Numeric"=431.0, "Numeric"=249.0}, {"Numeric"=438.0, "Numeric"=240.0}, {"Numeric"=448.0, "Numeric"=235.0}, {"Numeric"=455.0, "Numeric"=239.0}, {"Numeric"=457.0, "Numeric"=237.0}, {"Numeric"=449.0, "Numeric"=237.0}, {"Numeric"=446.0, "Numeric"=242.0}, {"Numeric"=425.0, "Numeric"=244.0}, {"Numeric"=402.0, "Numeric"=254.0}, {"Numeric"=378.0, "Numeric"=263.0}, {"Numeric"=355.0, "Numeric"=265.0}, {"Numeric"=334.0, "Numeric"=276.0}, {"Numeric"=313.0, "Numeric"=272.0}, {"Numeric"=292.0, "Numeric"=273.0}, {"Numeric"=285.0, "Numeric"=272.0}, {"Numeric"=260.0, "Numeric"=266.0}, {"Numeric"=263.0, "Numeric"=268.0}, {"Numeric"=262.0, "Numeric"=269.0}, {"Numeric"=264.0, "Numeric"=274.0}, {"Numeric"=274.0, "Numeric"=283.0}, {"Numeric"=286.0, "Numeric"=272.0}, {"Numeric"=305.0, "Numeric"=277.0}, {"Numeric"=326.0, "Numeric"=280.0}, {"Numeric"=354.0, "Numeric"=281.0}, {"Numeric"=380.0, "Numeric"=288.0}, {"Numeric"=397.0, "Numeric"=293.0}, {"Numeric"=384.0, "Numeric"=289.0}, {"Numeric"=409.0, "Numeric"=287.0}, {"Numeric"=406.0, "Numeric"=292.0}, {"Numeric"=399.0, "Numeric"=296.0}, {"Numeric"=384.0, "Numeric"=291.0}, {"Numeric"=367.0, "Numeric"=287.0}, {"Numeric"=354.0, "Numeric"=279.0}, {"Numeric"=346.0, "Numeric"=281.0}, {"Numeric"=335.0, "Numeric"=275.0}, {"Numeric"=322.0, "Numeric"=264.0}, {"Numeric"=313.0, "Numeric"=263.0}, {"Numeric"=298.0, "Numeric"=262.0}, {"Numeric"=287.0, "Numeric"=263.0}, {"Numeric"=274.0, "Numeric"=267.0}, {"Numeric"=266.0, "Numeric"=268.0}, {"Numeric"=254.0, "Numeric"=267.0}, {"Numeric"=252.0, "Numeric"=268.0}, {"Numeric"=225.0, "Numeric"=271.0}, {"Numeric"=232.0, "Numeric"=274.0}, {"Numeric"=261.0, "Numeric"=265.0}, {"Numeric"=268.0, "Numeric"=256.0}, {"Numeric"=257.0, "Numeric"=271.0}, {"Numeric"=264.0, "Numeric"=277.0}, {"Numeric"=264.0, "Numeric"=277.0}, {"Numeric"=331.0, "Numeric"=261.0}, {"Numeric"=333.0, "Numeric"=270.0}, {"Numeric"=335.0, "Numeric"=273.0}, {"Numeric"=336.0, "Numeric"=290.0}, {"Numeric"=344.0, "Numeric"=283.0}, {"Numeric"=353.0, "Numeric"=273.0}, {"Numeric"=353.0, "Numeric"=276.0}, {"Numeric"=353.0, "Numeric"=282.0}, {"Numeric"=358.0, "Numeric"=275.0}, {"Numeric"=362.0, "Numeric"=272.0}, {"Numeric"=370.0, "Numeric"=272.0}, {"Numeric"=371.0, "Numeric"=275.0}, {"Numeric"=398.0, "Numeric"=288.0}, {"Numeric"=420.0, "Numeric"=294.0}, {"Numeric"=430.0, "Numeric"=298.0}, {"Numeric"=423.0, "Numeric"=292.0}, {"Numeric"=421.0, "Numeric"=299.0}, {"Numeric"=406.0, "Numeric"=298.0}, {"Numeric"=404.0, "Numeric"=298.0}, {"Numeric"=385.0, "Numeric"=297.0}, {"Numeric"=383.0, "Numeric"=297.0}, {"Numeric"=377.0, "Numeric"=297.0}, {"Numeric"=376.0, "Numeric"=297.0}, {"Numeric"=372.0, "Numeric"=313.0}, {"Numeric"=366.0, "Numeric"=310.0}, {"Numeric"=375.0, "Numeric"=306.0}, {"Numeric"=384.0, "Numeric"=305.0}, {"Numeric"=396.0, "Numeric"=311.0}, {"Numeric"=402.0, "Numeric"=321.0}, {"Numeric"=455.0, "Numeric"=304.0}, {"Numeric"=456.0, "Numeric"=215.0}, {"Numeric"=443.0, "Numeric"=301.0}, {"Numeric"=423.0, "Numeric"=324.0}, {"Numeric"=411.0, "Numeric"=321.0}, {"Numeric"=399.0, "Numeric"=320.0}, {"Numeric"=392.0, "Numeric"=310.0}, {"Numeric"=385.0, "Numeric"=297.0}, {"Numeric"=358.0, "Numeric"=296.0}, {"Numeric"=351.0, "Numeric"=296.0}, {"Numeric"=335.0, "Numeric"=295.0}, {"Numeric"=330.0, "Numeric"=294.0}, {"Numeric"=323.0, "Numeric"=295.0}, {"Numeric"=323.0, "Numeric"=295.0}, {"Numeric"=411.0, "Numeric"=307.0}, {"Numeric"=412.0, "Numeric"=320.0}, {"Numeric"=415.0, "Numeric"=320.0}, {"Numeric"=416.0, "Numeric"=315.0}, {"Numeric"=415.0, "Numeric"=320.0}, {"Numeric"=409.0, "Numeric"=311.0}, {"Numeric"=408.0, "Numeric"=318.0}, {"Numeric"=405.0, "Numeric"=313.0}, {"Numeric"=401.0, "Numeric"=311.0}, {"Numeric"=401.0, "Numeric"=311.0}, {"Numeric"=394.0, "Numeric"=324.0}, {"Numeric"=396.0, "Numeric"=331.0}, {"Numeric"=405.0, "Numeric"=311.0}, {"Numeric"=380.0, "Numeric"=310.0}, {"Numeric"=361.0, "Numeric"=309.0}, {"Numeric"=361.0, "Numeric"=309.0}, {"Numeric"=381.0, "Numeric"=310.0}, {"Numeric"=383.0, "Numeric"=310.0}, {"Numeric"=409.0, "Numeric"=258.0}, {"Numeric"=417.0, "Numeric"=252.0}, {"Numeric"=421.0, "Numeric"=239.0}, {"Numeric"=420.0, "Numeric"=232.0}, {"Numeric"=423.0, "Numeric"=228.0}, {"Numeric"=424.0, "Numeric"=231.0}, {"Numeric"=421.0, "Numeric"=228.0}, {"Numeric"=417.0, "Numeric"=230.0}, {"Numeric"=404.0, "Numeric"=242.0}, {"Numeric"=404.0, "Numeric"=254.0}, {"Numeric"=403.0, "Numeric"=263.0}, {"Numeric"=405.0, "Numeric"=267.0}, {"Numeric"=421.0, "Numeric"=273.0}, {"Numeric"=423.0, "Numeric"=273.0}, {"Numeric"=423.0, "Numeric"=279.0}, {"Numeric"=424.0, "Numeric"=297.0}, {"Numeric"=403.0, "Numeric"=302.0}, {"Numeric"=406.0, "Numeric"=294.0}, {"Numeric"=394.0, "Numeric"=290.0}, {"Numeric"=380.0, "Numeric"=289.0}, {"Numeric"=361.0, "Numeric"=288.0}, {"Numeric"=358.0, "Numeric"=288.0}, {"Numeric"=356.0, "Numeric"=288.0}, {"Numeric"=353.0, "Numeric"=288.0}, {"Numeric"=334.0, "Numeric"=292.0}, {"Numeric"=334.0, "Numeric"=287.0}, {"Numeric"=332.0, "Numeric"=287.0}, {"Numeric"=332.0, "Numeric"=287.0}, {"Numeric"=352.0, "Numeric"=254.0}, {"Numeric"=362.0, "Numeric"=254.0}, {"Numeric"=377.0, "Numeric"=251.0}, {"Numeric"=389.0, "Numeric"=249.0}, {"Numeric"=411.0, "Numeric"=240.0}, {"Numeric"=419.0, "Numeric"=228.0}, {"Numeric"=433.0, "Numeric"=233.0}, {"Numeric"=423.0, "Numeric"=236.0}, {"Numeric"=427.0, "Numeric"=238.0}, {"Numeric"=427.0, "Numeric"=238.0}, {"Numeric"=433.0, "Numeric"=246.0}, {"Numeric"=438.0, "Numeric"=265.0}, {"Numeric"=441.0, "Numeric"=269.0}, {"Numeric"=441.0, "Numeric"=275.0}, {"Numeric"=440.0, "Numeric"=291.0}, {"Numeric"=448.0, "Numeric"=292.0}, {"Numeric"=451.0, "Numeric"=293.0}, {"Numeric"=457.0, "Numeric"=316.0}, {"Numeric"=454.0, "Numeric"=331.0}, {"Numeric"=441.0, "Numeric"=309.0}, {"Numeric"=434.0, "Numeric"=315.0}, {"Numeric"=436.0, "Numeric"=308.0}, {"Numeric"=427.0, "Numeric"=298.0}, {"Numeric"=423.0, "Numeric"=300.0}, {"Numeric"=406.0, "Numeric"=294.0}, {"Numeric"=398.0, "Numeric"=287.0}, {"Numeric"=391.0, "Numeric"=282.0}, {"Numeric"=384.0, "Numeric"=279.0}, {"Numeric"=377.0, "Numeric"=276.0}, {"Numeric"=369.0, "Numeric"=276.0}, {"Numeric"=368.0, "Numeric"=272.0}, {"Numeric"=364.0, "Numeric"=269.0}, {"Numeric"=364.0, "Numeric"=272.0}, {"Numeric"=354.0, "Numeric"=279.0}, {"Numeric"=348.0, "Numeric"=284.0}, {"Numeric"=344.0, "Numeric"=288.0}, {"Numeric"=340.0, "Numeric"=285.0}, {"Numeric"=340.0, "Numeric"=280.0}, {"Numeric"=343.0, "Numeric"=285.0}, {"Numeric"=345.0, "Numeric"=288.0}, {"Numeric"=355.0, "Numeric"=278.0}, {"Numeric"=354.0, "Numeric"=281.0}, {"Numeric"=358.0, "Numeric"=288.0}, {"Numeric"=356.0, "Numeric"=288.0}, {"Numeric"=394.0, "Numeric"=268.0}, {"Numeric"=368.0, "Numeric"=266.0}, {"Numeric"=369.0, "Numeric"=267.0}, {"Numeric"=350.0, "Numeric"=266.0}, {"Numeric"=386.0, "Numeric"=265.0}, {"Numeric"=386.0, "Numeric"=265.0}]
  out "Number of Frames":u32
  out "Image 3":T2(plugin-control)
  in  "Reference Points":T3
  in  "AVI Path":path=path "E:/PhD work/PhD research work/Videos/Chen Jin vs Hu Yun (Edited).avi"
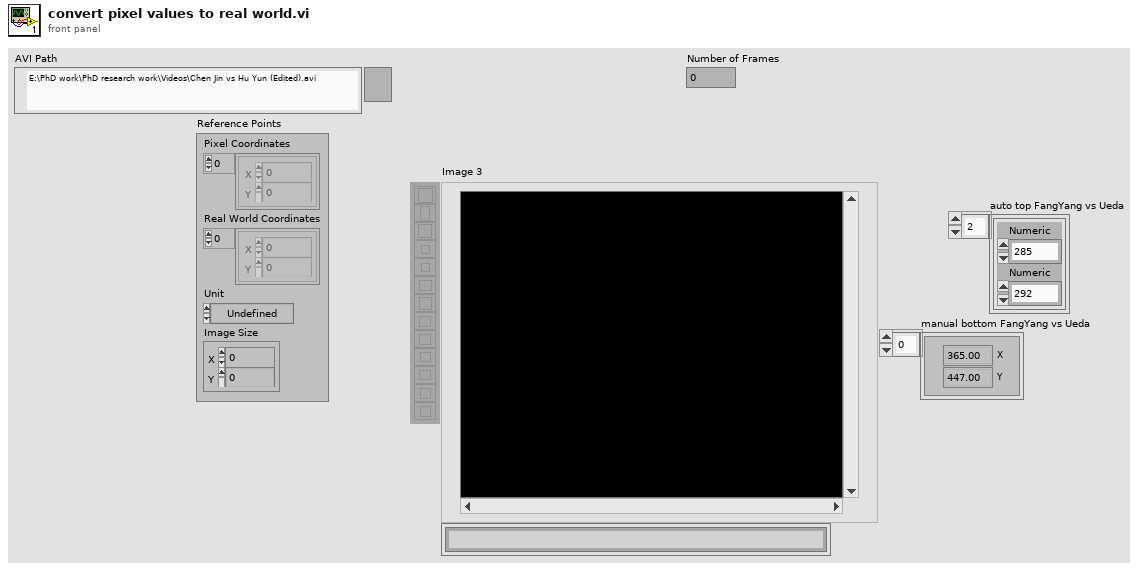
[diagram p1: front panel]
types:
  T1 = typedef "IMAQ Point" = cluster{"X":sgl, "Y":sgl}
  T2 = typedef "IMAQ Image.ctl" = refnum<image>
  T3 = typedef "Calibration Reference Points.ctl" = cluster{"Pixel Coordinates":cluster{"X":dbl, "Y":dbl}[], "Real World Coordinates":cluster{"X":dbl, "Y":dbl}[], "Unit":T4, "Image Size":cluster{"X":u32, "Y":u32}}
  T4 = typedef "Image Unit" = enum32{"Undefined", "Angström", "Micrometer", "Millimeter", "Centimeter", "Meter", "Kilometer", "Microinch", "Inch", "Feet", "Nautical miles", "Standard miles", "Steps"}
  T5 = cluster{"Origin Pixel":cluster{"X":sgl, "Y":sgl}, "Angle Relative to Horizontal (deg)":sgl, "Axis Reference":u32}
  T6 = typedef "Image Type" = u32
  T7 = typedef "AviRefnum.ctl" = refnum<k1>
  T8 = cluster{"width":u32, "height":u32, "framesPerSecond":u32, "compressionFilter":string, "hasData":bool}
  T9 = cluster{cluster{u32, u32}[], cluster{u32, u32}[], "Unit":u32}
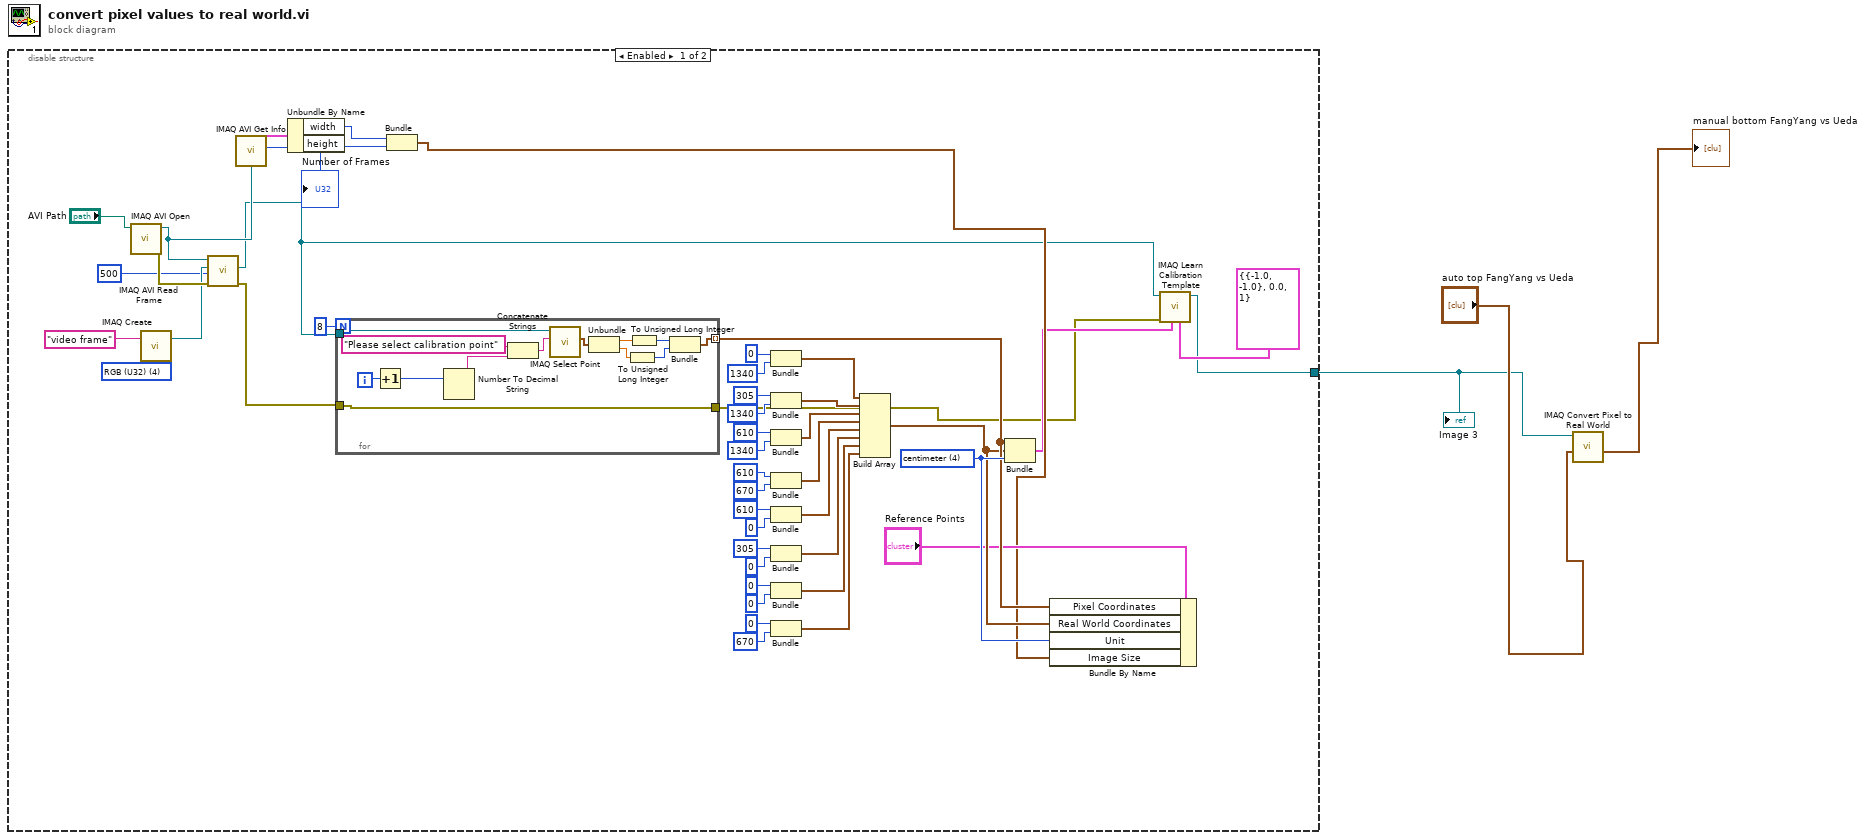
[diagram p0: block diagram]
diagram:
  n1 = disable-structure shown="Enabled" {
    disable-tunnel: [w4 _] -> w1
    frame Enabled {
      w15 = u32 4 items=["Undefined", "Angstrom", "micrometer", "millimeter", "centimeter", "meter", "kilometer", "microinch", "inch", "feet", "nautic miles", "standard miles", "steps"] ("Unit")
      w49 = T6 4 items=["Grayscale (U8)", "Grayscale (I16)", "Grayscale (SGL)", "Complex (CSG)", "RGB (U32)", "HSL (U32)", "RGB (U64)", "Grayscale (U16)"] ("Image Type")
      n2 = call "IMAQ AVI Open"("AVI Path"="AVI Path") -> ("error out"=w47:errorcluster, "Avi Refnum"=w44:T7)  [unwired: 9 in]
      n3 = call "IMAQ Create"("Image Name"="video frame", "Image Type"=w49) -> ("New Image"=w46:T2)  [unwired: 3 in, 1 out]
      n4 = call "IMAQ AVI Read Frame"("error in (no error)"=w47, "Frame Number"=u32 500, "Image"=w46, "Avi Refnum"=w44) -> ("error out"=w10:errorcluster, "Image Out"=w7:T2)  [unwired: 4 in, 2 out]
      n5 = call "IMAQ AVI Get Info"("Avi Refnum"=w44) -> ("Number of Frames"=→"Number of Frames":u32, "Frame Data"=w43:T8)  [unwired: 6 in, 3 out]
      n6 = Unbundle By Name(w43) -> ("width"=w42:u32, "height"=w41:u32)
      n7 = for {
        N: 8 -> [_]
        tunnel: w7 -> [w63]
        tunnel: [w52] -> w14 mode=indexing
        tunnel: w10 -> [w51]
        tunnel: [w51] -> w5
        i -> [w62]
        n8 = Increment(x=w62) -> (x+1=w59:i32)
        n9 = Number To Decimal String(number=w59) -> (decimal integer string=w58:string)  [unwired: 1 in]
        n10 = Concatenate Strings("Please select calibration point" ("string"), w58) -> (w60:string)
        n11 = call "IMAQ Select Point"("Prompt"=w60, "Image In"=w63) -> ("Point"=w57:T1)  [unwired: 6 in, 3 out]
        n12 = Unbundle(w57) -> ("X"=w56:sgl, "Y"=w55:sgl)
        n13 = To Unsigned Long Integer(number=w55) -> (unsigned 32bit integer=w54:u32)
        n14 = To Unsigned Long Integer(number=w56) -> (unsigned 32bit integer=w53:u32)
        n15 = Bundle(w53, w54) -> (w52:cluster{u32, u32})  [unwired: 1 in]
      }
      n16 = Bundle("width"=w42, "height"=w41) -> (w11:cluster{"width":u32, "height":u32})  [unwired: 1 in]
      n17 = Bundle(u32 0, u32 1340) -> (w18:cluster{u32, u32})  [unwired: 1 in]
      n18 = Bundle(u32 305, u32 1340) -> (w33:cluster{u32, u32})  [unwired: 1 in]
      n19 = Bundle(u32 610, u32 1340) -> (w34:cluster{u32, u32})  [unwired: 1 in]
      n20 = Bundle(u32 610, u32 670) -> (w35:cluster{u32, u32})  [unwired: 1 in]
      n21 = Bundle(u32 610, u32 0) -> (w36:cluster{u32, u32})  [unwired: 1 in]
      n22 = Bundle(u32 305, u32 0) -> (w37:cluster{u32, u32})  [unwired: 1 in]
      n23 = Bundle(u32 0, u32 0) -> (w38:cluster{u32, u32})  [unwired: 1 in]
      n24 = Bundle(u32 0, u32 670) -> (w39:cluster{u32, u32})  [unwired: 1 in]
      n25 = Build Array(w18, w33, w34, w35, w36, w37, w38, w39) -> (w13:cluster{u32, u32}[])
      n26 = Bundle(w14, w13, "Unit"=w15) -> (w8:T9)  [unwired: 1 in]
      n27 = Bundle By Name(cluster="Reference Points", "Pixel Coordinates"=w14, "Real World Coordinates"=w13, "Unit"=w15, "Image Size"=w11) -> ()  [unwired: 1 out]
      n28 = call "IMAQ Learn Calibration Template"("Calibration Axis Info"=T5 {"Origin Pixel"={"X"=-1.0, "Y"=-1.0}, "Angle Relative to Horizontal (deg)"=0.0, "Axis Reference"=1}, "Reference Points"=w8, "error in (no error)"=w5, "Image"=w7) -> ("Calibrated Image"=w4:T2)  [unwired: 5 in, 2 out]
    }
    frame Disabled {
    }
  }
  "Image 3" <- w1
  n29 = call "IMAQ Convert Pixel to Real World"("Array of Pixel Coordinates"="auto top FangYang vs Ueda", "Calibrated Image"=w1) -> ("Array of Real World Coordinates"=→"manual bottom FangYang vs Ueda":cluster{"X":sgl, "Y":sgl}[])  [unwired: 4 in, 5 out]
